vi "Write FolderName to Crypt.vi"(8 "error in (no error)":errorcluster, 10 "FolderName to Crypt":path, 11 "Crypter in":refnum<class "Crypter.lvclass">) -> (0 "error out":errorcluster, 3 "Crypter out":refnum<class "Crypter.lvclass">)   [LabVIEW 2016, in "Crypter.lvclass"]
uses:
  Crypter.lvclass
  Crypter.lvclass/Crypter.ctl
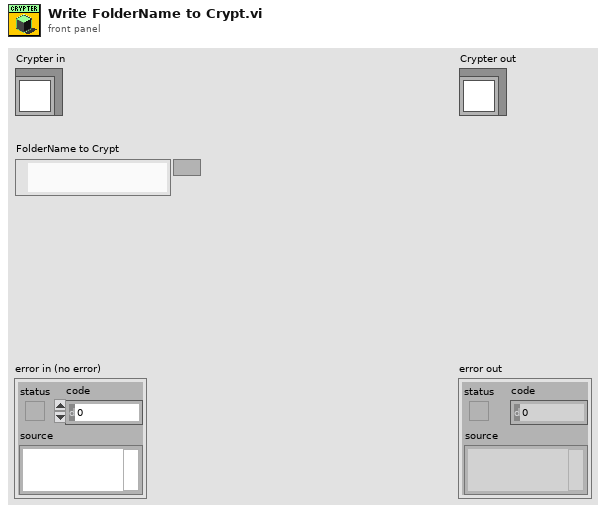
[diagram p1: front panel]
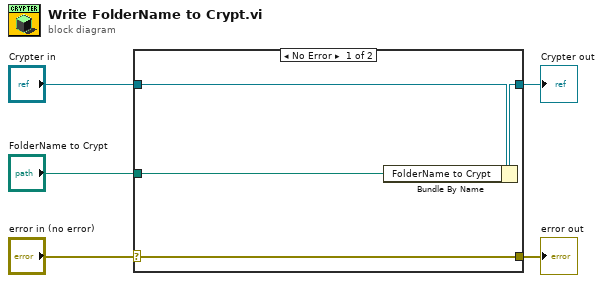
[diagram p0: block diagram]
diagram:
  n1 = case shown="No Error" "error in (no error)" {
    selector: "error in (no error)" -> [w9 w10]
    tunnel: [w9 w10] -> w4
    tunnel: [w7 w11] -> w2
    tunnel: "Crypter in" -> [w8 w11]
    tunnel: "FolderName to Crypt" -> [w6 _]
    frame No Error {
      n2 = Bundle By Name(cluster=w8, "FolderName to Crypt"=w6) -> (w7:refnum<class "Crypter.lvclass">)
    }
    frame Error {
    }
  }
  "error out" <- w4
  "Crypter out" <- w2
